vi "Arm State Machine Test.vi"() -> ()   [LabVIEW 2015]
uses:
  Intake States.ctl
  Arm States.ctl
panel:
  out "State":string
  out "Enum":T1
  in  "Arm On Target":bool
  in  "Shoot Button":bool
  in  "Intake State":T2
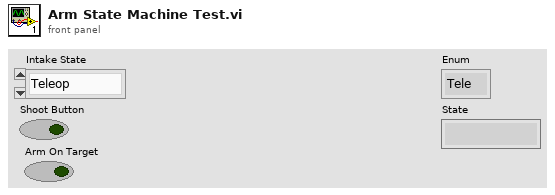
[diagram p1: front panel]
types:
  T1 = typedef "Arm States.ctl" = enum16{"Tele", "Aim", "Outtake", "Rev Up", "Shoot"}
  T2 = typedef "Intake States.ctl" = enum16{"Teleop", "Centering In", "Centering Out"}
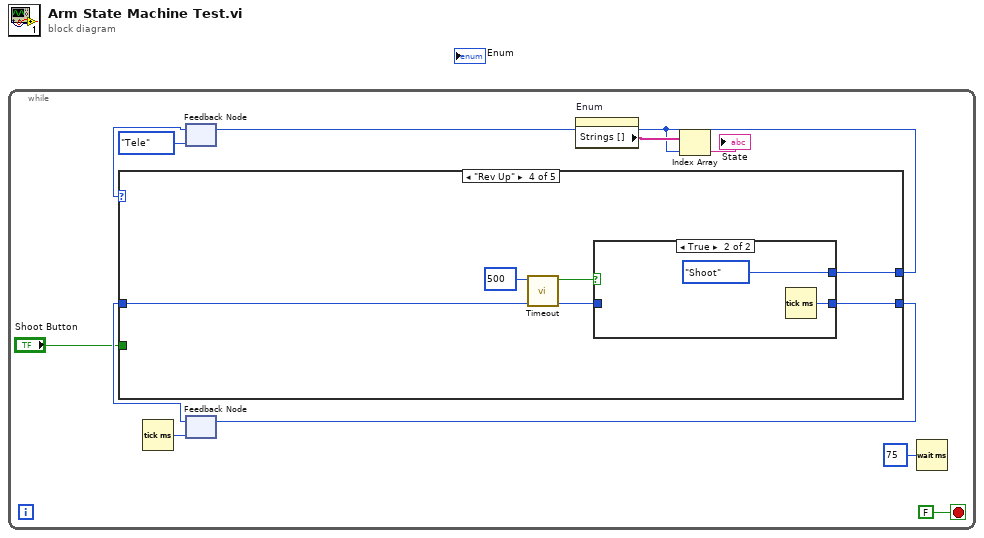
[diagram p0: block diagram]
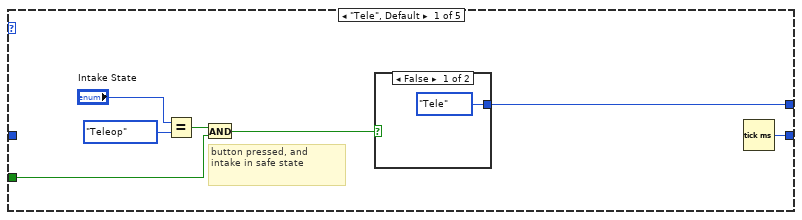
[diagram p2: hidden frame]
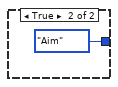
[diagram p3: hidden frame]
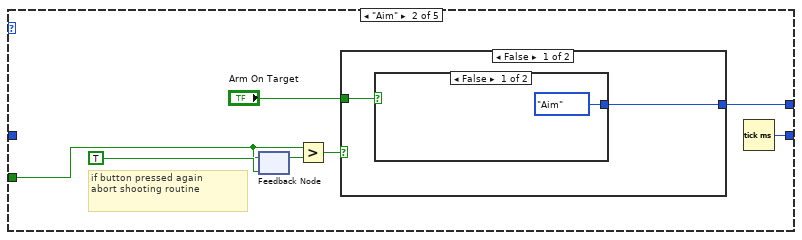
[diagram p4: hidden frame]
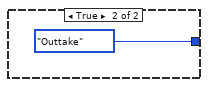
[diagram p5: hidden frame]
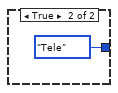
[diagram p6: hidden frame]
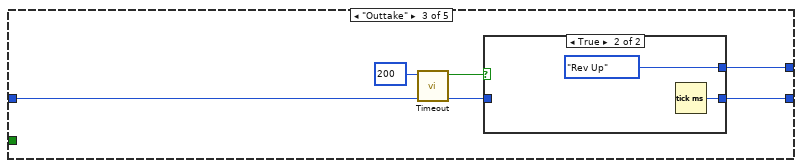
[diagram p7: hidden frame]
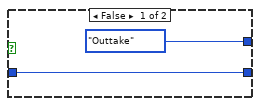
[diagram p8: hidden frame]
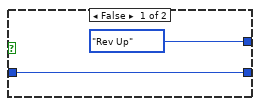
[diagram p9: hidden frame]
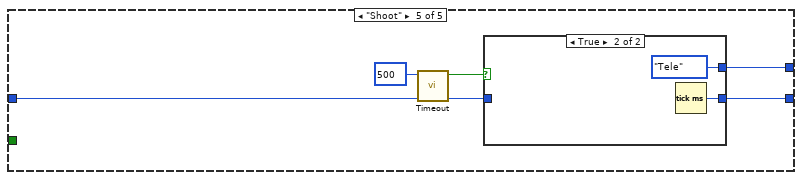
[diagram p10: hidden frame]
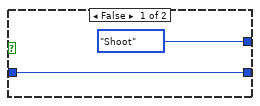
[diagram p11: hidden frame]
diagram:
  n1 = while {
    stop <- FALSE stop-if-true
    n2 = Tick Count (ms)() -> (millisecond timer value=w10:u32)
    n3 = feedback #1(Arm_States."Tele" ("Enum")) -> (w9:T1)
    n4 = feedback #2(w10) -> (w8:u32)
    n5 = case shown="\"Rev Up\"" w9 {
      tunnel: w8 -> [_ _ w37 w47 w57]
      tunnel: [w18 w27 w34 w44 w54] -> w5
      tunnel: [w17 w26 w35 w45 w55] -> w1
      tunnel: "Shoot Button" -> [w12 w24 _ _ _]
      frame "Tele", Default {
        # "button pressed, and\nintake in safe state"
        n6 = Equal?(x="Intake State", y=Intake_States."Teleop") -> (x = y?=w15:bool)
        n7 = And(x=w15, y=w12) -> (x .and. y?=w14:bool)
        n8 = case shown="False" w14 {
          tunnel: [Arm_States."Tele" ("Enum") Arm_States."Aim" ("Enum")] -> w17
          frame False {
          }
          frame True {
          }
        }
        n9 = Tick Count (ms)() -> (millisecond timer value=w18:u32)
      }
      frame "Aim" {
        # "if button pressed again\nabort shooting routine"
        n10 = feedback-in #3(w24) -> ()
        n11 = feedback #3(TRUE) -> (w23:bool)
        n12 = Greater?(x=w24, y=w23) -> (0:w22:bool)
        n13 = case shown="False" w22 {
          tunnel: [w29 Arm_States."Tele" ("Enum")] -> w26
          tunnel: "Arm On Target" -> [w28 _]
          frame False {
            n14 = case shown="False" w28 {
              tunnel: [Arm_States."Aim" ("Enum") Arm_States."Outtake" ("Enum")] -> w29
              frame False {
              }
              frame True {
              }
            }
          }
          frame True {
          }
        }
        n15 = Tick Count (ms)() -> (millisecond timer value=w27:u32)
      }
      frame "Outtake" {
        n16 = call "Timeout.vi"("Start Time In"=w37, "Time Limit"=u32 200 ("milliseconds to wait")) -> ("Start Time Out"=w33:u32, "Timeout"=w36:bool)  [unwired: 8 in]
        n17 = case shown="True" w36 {
          tunnel: [Arm_States."Outtake" ("Enum") Arm_States."Rev Up" ("Enum")] -> w35
          tunnel: [w39 w41] -> w34
          tunnel: w33 -> [w39 _]
          frame False {
          }
          frame True {
            n18 = Tick Count (ms)() -> (millisecond timer value=w41:u32)
          }
        }
      }
      frame "Rev Up" {
        n19 = call "Timeout.vi"("Start Time In"=w47, "Time Limit"=u32 500 ("milliseconds to wait")) -> ("Start Time Out"=w43:u32, "Timeout"=w46:bool)  [unwired: 8 in]
        n20 = case shown="True" w46 {
          tunnel: [Arm_States."Rev Up" ("Enum") Arm_States."Shoot" ("Enum")] -> w45
          tunnel: [w49 w51] -> w44
          tunnel: w43 -> [w49 _]
          frame False {
          }
          frame True {
            n21 = Tick Count (ms)() -> (millisecond timer value=w51:u32)
          }
        }
      }
      frame "Shoot" {
        n22 = call "Timeout.vi"("Start Time In"=w57, "Time Limit"=u32 500 ("milliseconds to wait")) -> ("Start Time Out"=w53:u32, "Timeout"=w56:bool)  [unwired: 8 in]
        n23 = case shown="True" w56 {
          tunnel: [Arm_States."Shoot" ("Enum") Arm_States."Tele" ("Enum")] -> w55
          tunnel: [w59 w61] -> w54
          tunnel: w53 -> [w59 _]
          frame False {
          }
          frame True {
            n24 = Tick Count (ms)() -> (millisecond timer value=w61:u32)
          }
        }
      }
    }
    n25 = feedback-in #1(w1) -> ()
    n26 = feedback-in #2(w5) -> ()
    n27 = property on="Enum" class="Enum (strict)"() -> ("Strings []"=w6:string[])  [unwired: 2 in, 2 out]
    n28 = Index Array(array=w6, index=w1) -> (element=→"State":string)
    n29 = Wait (ms)(milliseconds to wait=u32 75) -> ()  [unwired: 1 out]
  }
